vi "DB_创建Temperature表.vi"(8 "error in (no error)":errorcluster caption="错误输入（无错误）") -> (0 "error out":errorcluster caption="错误输出", 3 "SQLite Connection":refnum<class "Connection.lvclass">)   [LabVIEW 2018]
uses:
  <vilib>/drjdpowell/SQLite Library/SQL Connection/Connection.lvclass
  <vilib>/Utility/sysdir.llb/System Directory Type.ctl
  <vilib>/drjdpowell/SQLite Library/SQL Connection/Open (path).vi
  <vilib>/drjdpowell/SQLite Library/SQL Connection/Open (string).vi
  <vilib>/AdvancedString/Path To Command Line String.vi
  <vilib>/drjdpowell/SQLite Library/SQL Connection/Execute SQL (No results).vi
  <vilib>/drjdpowell/SQLite Library/SQLite.lvlib
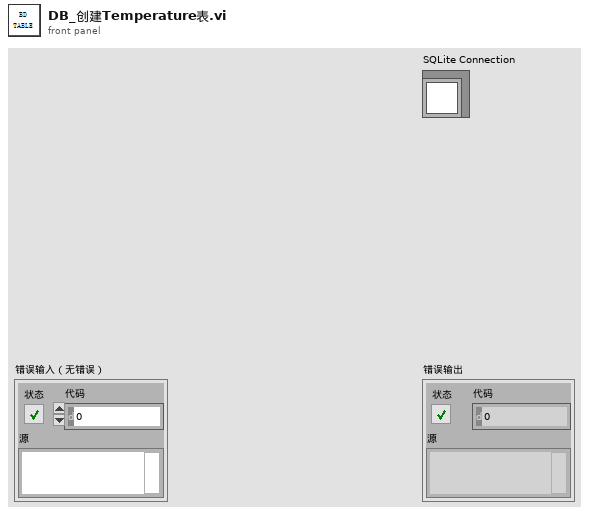
[diagram p1: front panel]
types:
  T1 = enum16{"New or existing", "Existing", "Read only"}
  T2 = typedef "System Directory Type.ctl" = i32
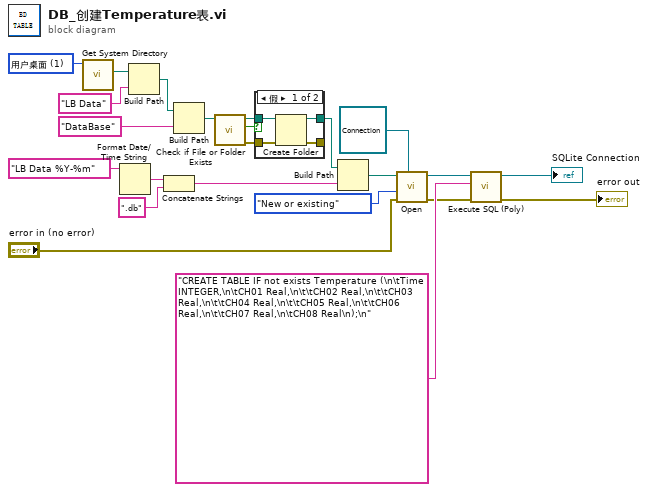
[diagram p0: block diagram]
diagram:
  w22 = T2 1 items=["用户目录"=0, "用户桌面"=1, "用户文档"=2, "用户应用程序数据"=3, "用户设置"=4, "用户临时目录"=5, "公共文档"=6, "公共应用程序数据"=7, "公共设置"=8, "公共缓存"=13, "系统核心库"=9, "系统安装库"=10, "应用程序文件"=11, "启动盘根目录"=12] ("system directory type")
  n1 = call <vilib>:"Get System Directory.vi"("system directory type"=w22) -> ("system directory"=w21:path)  [unwired: 10 in]
  n2 = Format Date/Time String(time format string (%c)="LB Data %Y-%m" ("时间格式字符串(%c)")) -> (date/time string=w9:string)  [unwired: 2 in]
  n3 = Build Path(base path=w21, name or relative path="LB Data" ("名称或相对路径")) -> (appended path=w15:path)
  n4 = Concatenate Strings(w9, ".db" ("时间格式字符串(%c)")) -> (w7:string)
  n5 = Build Path(base path=w15, name or relative path="DataBase" ("名称或相对路径")) -> (appended path=w11:path)
  n6 = call <vilib>:"Check if File or Folder Exists.vi"("path"=w11) -> ("error out"=w13:errorcluster, "file or folder exists?"=w14:bool, "dup path"=w12:path)  [unwired: 8 in]
  n7 = case shown="假" w14 {
    tunnel: w12 -> [w27 w28]
    tunnel: w13 -> [w26 w29]
    tunnel: [w25 w29] -> _
    tunnel: [w24 w28] -> w8
    frame False {
      n8 = Create Folder(path (use dialog)=w27, error in=w26) -> (created path=w24:path, error out=w25:errorcluster)  [unwired: 1 in, 1 out]
    }
    frame True {
    }
  }
  n9 = Build Path(base path=w8, name or relative path=w7) -> (appended path=w6:path)
  n10 = call-poly <vilib>:"Open.vi"("SQLite Connection type"=refnum<class "Connection.lvclass"> refnum, "error in (no error)"="error in (no error)", "File Option"=T1."New or existing", "db file"=w6) -> ("error out"=w2:errorcluster, "SQLite Connection"=w5:refnum<class "Connection.lvclass">)  [unwired: 6 in]
  n11 = call-poly <vilib>:"Execute SQL (Poly).vi"("error in (no error)"=w2, "SQL"="CREATE TABLE IF not exists Temperature (\n\tTime INTEGER,\n\tCH01 Real,\n\t\tCH02 Real,\n\t\tCH03 Real,\n\t\tCH04 Real,\n\t\tCH05 Real,\n\t\tCH06 Real,\n\t\tCH07 Real,\n\tCH08 Real\n);\n", "SQLite Connection in"=w5) -> ("error out"=→"error out":errorcluster, "SQLite Connection"=→"SQLite Connection":refnum<class "Connection.lvclass">)  [unwired: 7 in]
